vi "Read freq ref.vi"(8 "error in (no error)":errorcluster caption="에러 입력(에러 없음)", 11 "Haptic IC 입력":refnum<class "Haptic IC.lvclass">) -> (0 "error out":errorcluster caption="에러 출력", 2 "freq ref":refnum<vi>, 3 "Haptic IC 출력":refnum<class "Haptic IC.lvclass">)   [LabVIEW 2020, in "Haptic IC.lvclass"]
uses:
  Haptic IC.lvclass
  Haptic IC.lvclass/Haptic IC.ctl
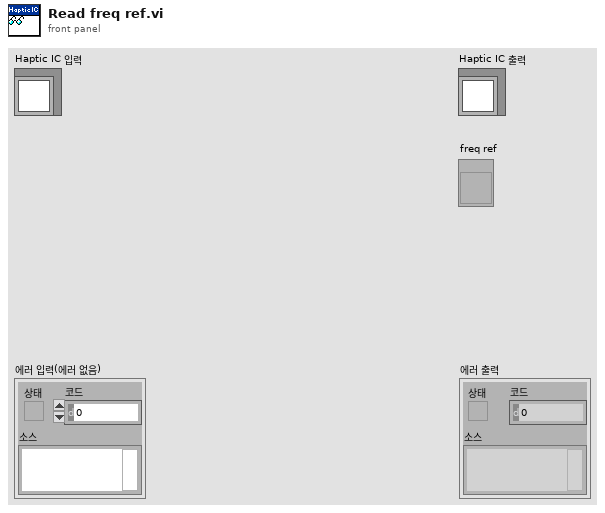
[diagram p1: front panel]
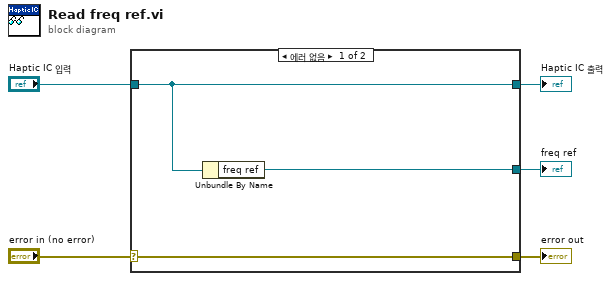
[diagram p0: block diagram]
diagram:
  n1 = case shown="에러 없음" "error in (no error)" {
    selector: "error in (no error)" -> [w8 w9]
    tunnel: [w8 w9] -> w4
    tunnel: [w7 w10] -> w2
    tunnel: "Haptic IC 입력" -> [w7 w10]
    tunnel: [w6 _] -> w1
    frame No Error {
      n2 = Unbundle By Name(w7) -> ("freq ref"=w6:refnum<vi>)
    }
    frame Error {
    }
  }
  "error out" <- w4
  "Haptic IC 출력" <- w2
  "freq ref" <- w1
